vi "Robot Global Data.vi"() -> ()   [LabVIEW 2011]
doc: "This global VI can contain as many global variables as you need. Place a control on the panel, give it a good name. To read or write to it from a VI, drag the icon to the diagram of that VI. You can also drag from the project. Click on the node to change which global you access. You shouldn't have multiple locations writing to a global or it will cause a race-condition."
uses:
  Robot Ctl.ctl
panel:
  in  "Firing Interval":dbl
  in  "Robot":T1
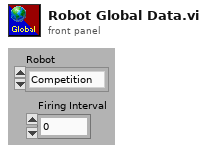
[diagram p1: front panel]
types:
  T1 = typedef "Robot Ctl.ctl" = enum16{"Competition", "Practice"}
diagram:
